vi "_isOverflowAllowed.vi"(11 "VariantBuffer in":refnum<class "VariantBuffer.lvclass">) -> (2 "Allow Overflow?":bool)   [LabVIEW 2013, in "CircularBuffer.lvlib" / "VariantBuffer.lvclass"]
uses:
  VariantBuffer.lvclass
  VariantBuffer.lvclass/VariantBuffer.ctl
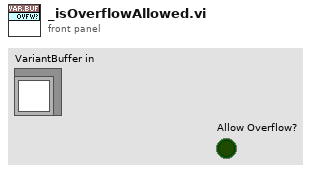
[diagram p1: front panel]
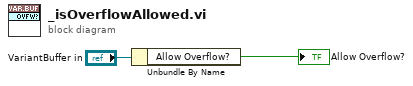
[diagram p0: block diagram]
diagram:
  n1 = Unbundle By Name("VariantBuffer in") -> ("Allow Overflow?"=→"Allow Overflow?":bool)
